vi "Host_9.vi"() -> ()   [LabVIEW 2020]
panel:
  in  "stop":bool
  out "Dane":waveform(dbl)(graph)
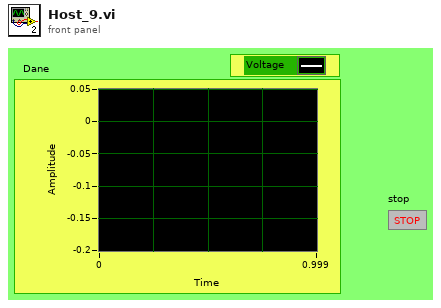
[diagram p1: front panel]
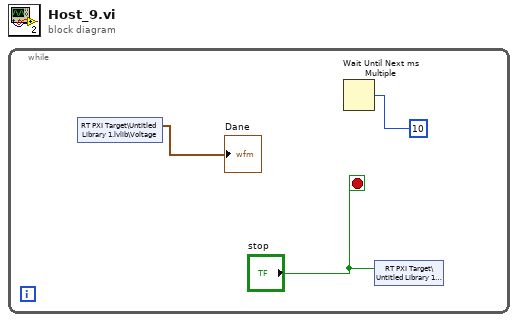
[diagram p0: block diagram]
diagram:
  n1 = while {
    stop <- "stop" stop-if-true
    n2 = shared-variable "RT PXI Target\\Untitled Library 1.lvlib\\Voltage"() -> (→"Dane":waveform(dbl))  [unwired: 1 in, 1 out]
    n3 = Wait Until Next ms Multiple(millisecond multiple=u32 10) -> ()  [unwired: 1 out]
    n4 = shared-variable "RT PXI Target\\Untitled Library 1.lvlib\\Stop"("stop") -> ()  [unwired: 1 in, 1 out]
  }
